vi "Close Output Session.vi"(8 "error in (no error)":errorcluster, 11 "PXI 8513 in":refnum<class "PXI 8513.lvclass">) -> (0 "error out":errorcluster, 3 "PXI 8513 out":refnum<class "PXI 8513.lvclass">)   [LabVIEW 2021, in "CAN.lvlib" / "PXI 8513.lvclass"]
uses:
  PXI 8513.lvclass
  PXI 8513.lvclass/PXI 8513.ctl
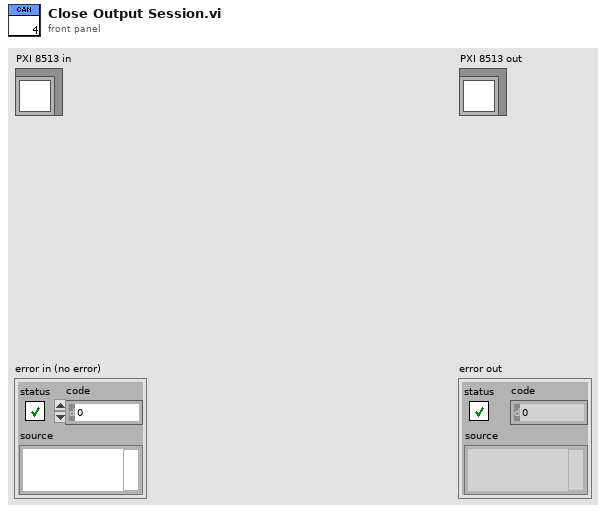
[diagram p1: front panel]
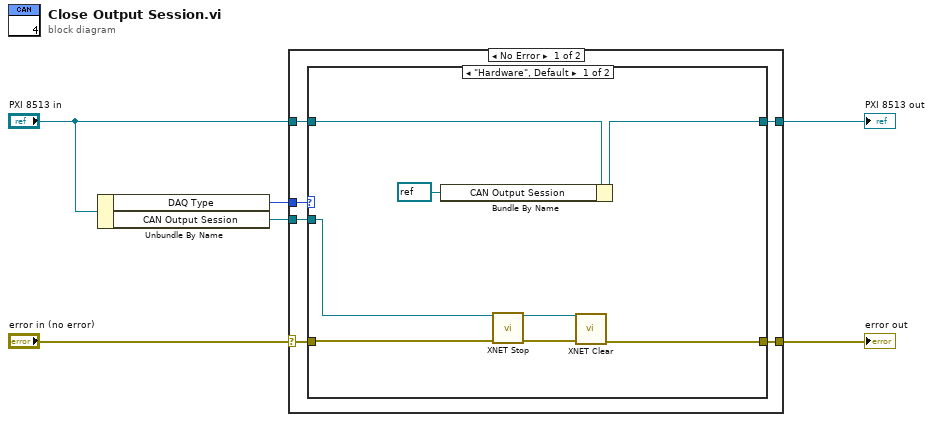
[diagram p0: block diagram]
diagram:
  n1 = Unbundle By Name("PXI 8513 in") -> ("DAQ Type"=w3:enum16{"Hardware", "Simulation"}, "CAN Output Session"=w2:refnum<k21>)
  n2 = case shown="No Error" "error in (no error)" {
    selector: "error in (no error)" -> [w10 w23]
    tunnel: [w8 w24] -> w5
    tunnel: "PXI 8513 in" -> [w12 w24]
    tunnel: w3 -> [w11 _]
    tunnel: w2 -> [w9 _]
    tunnel: [w7 w23] -> w1
    frame No Error {
      n3 = case shown="\"Hardware\", Default" w11 {
        tunnel: w12 -> [w16 w21]
        tunnel: w10 -> [w18 w22]
        tunnel: w9 -> [w17 _]
        tunnel: [w14 w21] -> w8
        tunnel: [w15 w22] -> w7
        frame "Hardware", Default {
          n4 = Bundle By Name(cluster=w16, "CAN Output Session"=refnum<k21> refnum ("Output.CAN Output Session")) -> (w14:refnum<class "PXI 8513.lvclass">)
          n5 = call <vilib>:"XNET Stop.vi"("session in"=w17, "error in (no error)"=w18) -> ("session out"=w20:refnum<k21>, "error out"=w19:errorcluster)  [unwired: 12 in]
          n6 = call <vilib>:"XNET Clear.vi"("session in"=w20, "error in (no error)"=w19) -> ("error out"=w15:errorcluster)  [unwired: 13 in]
        }
        frame "Simulation" {
        }
      }
    }
    frame Error {
    }
  }
  "error out" <- w1
  "PXI 8513 out" <- w5
